vi "calibrateValue.vi"(8 "error in (no error)":errorcluster, 10 "value":string, 11 "DigitalChannel in":refnum<class "DigitalChannel.lvclass">) -> (0 "error out":errorcluster, 2 "calibratedValue":dbl, 3 "DigitalChannel out":refnum<class "DigitalChannel.lvclass">)   [LabVIEW 2009, in "Tools.lvlib" / "DatabaseHelpers.lvlib" / "DigitalChannel.lvclass"]
uses:
  DigitalChannel.lvclass
  DigitalChannel.lvclass/DigitalChannel.ctl
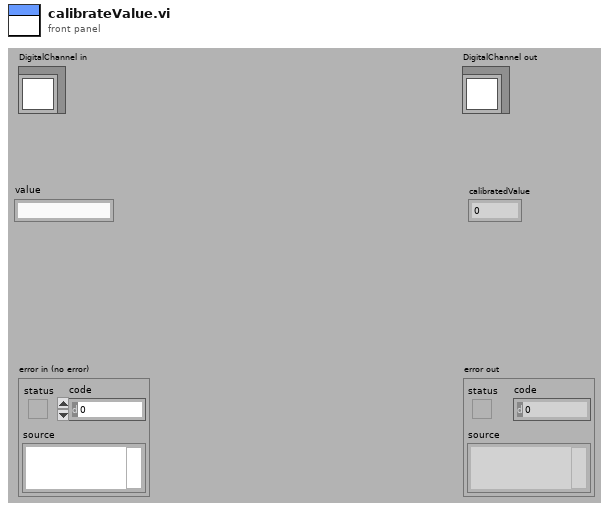
[diagram p1: front panel]
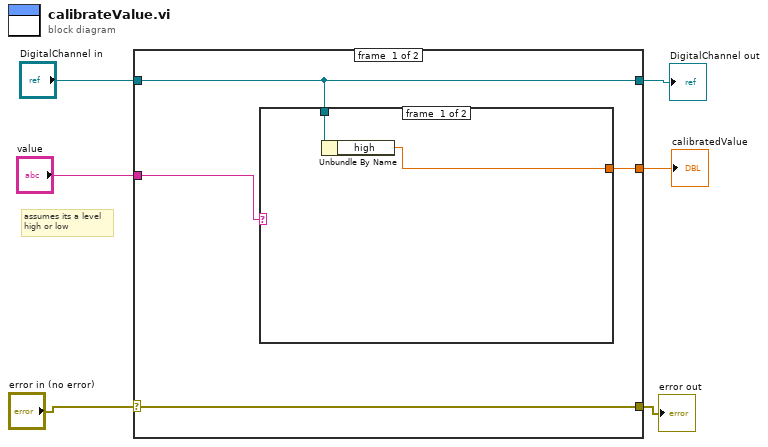
[diagram p0: block diagram]
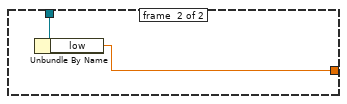
[diagram p2: hidden frame]
diagram:
  # "assumes its a level\nhigh or low"
  n1 = case shown="No Error" "error in (no error)" {
    selector: "error in (no error)" -> [w10 w15]
    tunnel: "DigitalChannel in" -> [w9 w16]
    tunnel: [w9 w16] -> w5
    tunnel: [w10 w15] -> w3
    tunnel: "value" -> [w7 _]
    tunnel: [w8 _] -> w1
    frame #0 {
      n2 = case shown="\"high\", Default" w7 {
        tunnel: w9 -> [w12 w14]
        tunnel: [w11 w13] -> w8
        frame #0 {
          n3 = Unbundle By Name(w12) -> ("high"=w11:dbl)
        }
        frame #1 {
          n4 = Unbundle By Name(w14) -> ("low"=w13:dbl)
        }
      }
    }
    frame #1 {
    }
  }
  "error out" <- w3
  "DigitalChannel out" <- w5
  "calibratedValue" <- w1
